vi "检查并创建文件夹.vi"(9 "error in (no error)":errorcluster caption="错误输入（无错误）", 10 "路径in":path) -> (1 "error out":errorcluster, 2 "dup path":path)   [LabVIEW 2020]
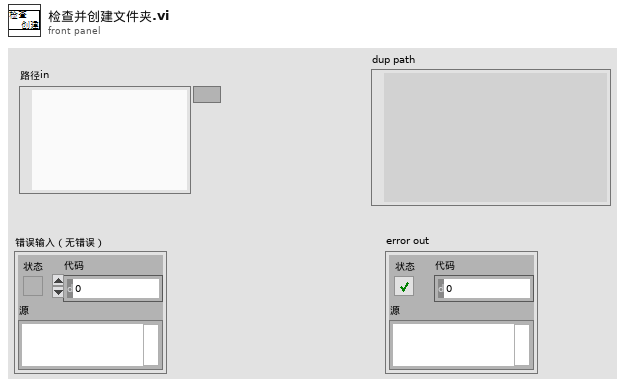
[diagram p1: front panel]
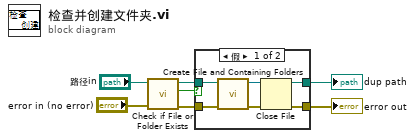
[diagram p0: block diagram]
diagram:
  n1 = call <vilib>:"Check if File or Folder Exists.vi"("error in (no error)"="error in (no error)", "path"="路径in") -> ("error out"=w4:errorcluster, "file or folder exists?"=w6:bool, "dup path"=w5:path)  [unwired: 7 in]
  n2 = case shown="假" w6 {
    tunnel: w5 -> [w13 w15]
    tunnel: w4 -> [w12 w14]
    tunnel: [w9 w15] -> w3
    tunnel: [w8 w14] -> w2
    frame False {
      n3 = call <vilib>:"Create File and Containing Folders.vi"("error in (no error)"=w12, "file path"=w13) -> ("error out"=w11:errorcluster, "refnum out"=w10:refnum<file>)  [unwired: 8 in]
      n4 = Close File(refnum=w10, error in=w11) -> (path=w9:path, error out=w8:errorcluster)
    }
    frame True {
    }
  }
  "dup path" <- w3
  "error out" <- w2
